vi "Config.Deploy Config Files.vi"(8 "error in (no error)":errorcluster, 11 "Install Config Items":T1[](array[typedef])) -> (0 "error out":errorcluster)   [LabVIEW 2018]
uses:
  Config.Install File Item.ctl
  <vilib>/KATE/Files/File Utils.lvlib
panel:
  # "This VI copies a file or folder from one location to another on the PC.\nFiles/Folders will only be copied of they do not exist."
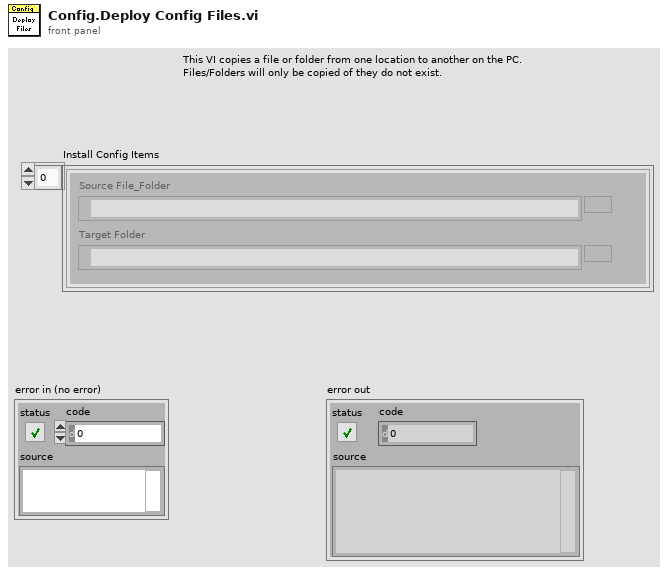
[diagram p1: front panel]
types:
  T1 = typedef "Config.Install File Item.ctl" = cluster{"Source File_Folder":path, "Target Folder":path}
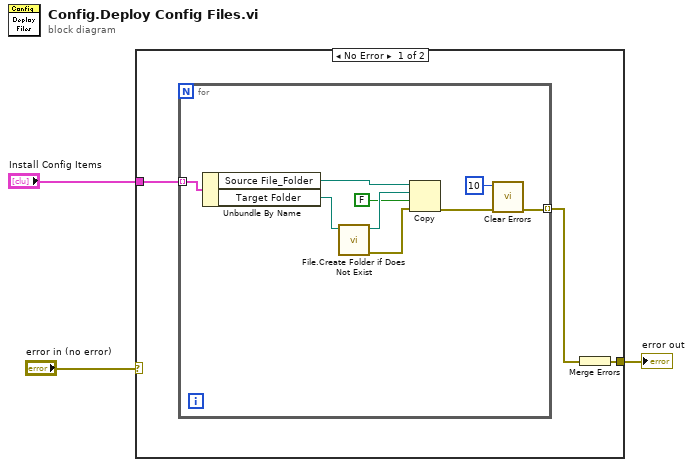
[diagram p0: block diagram]
diagram:
  n1 = case shown="No Error" "error in (no error)" {
    selector: "error in (no error)" -> [_ w16]
    tunnel: "Install Config Items" -> [w6 _]
    tunnel: [w4 w16] -> w1
    frame No Error {
      n2 = for {
        tunnel: w6 -> [w15] mode=indexing
        tunnel: [w8] -> w5 mode=indexing
        n3 = Unbundle By Name(w15) -> ("Source File_Folder"=w14:path, "Target Folder"=w13:path)
        n4 = call <vilib>:"File.Create Folder if Does Not Exist.vi"("Path"=w13) -> ("error out"=w11:errorcluster, "Dup Path"=w12:path)  [unwired: 8 in, 1 out]
        n5 = Copy(8:w11, 9:FALSE ("overwrite (F)"), 10:w12, 11:w14) -> (0:w9:errorcluster)  [unwired: 1 in, 2 out]
        n6 = call <vilib>:"Clear Errors.vi"("error in (no error)"=w9, "specific error code to clear (0: all)"=10) -> ("error out"=w8:errorcluster)  [unwired: 4 in, 1 out]
      }
      n7 = Merge Errors(w5) -> (w4:errorcluster)
    }
    frame Error {
    }
  }
  "error out" <- w1
